vi "C to F.vi"(11 "Celsius":dbl) -> (3 "Fahrenheit":dbl)   [LabVIEW 2023, in "Simple Dual Mode Thermometer XControl.xctl"]
doc: "This VI converts degrees Celsius to degrees Fahrenheit."
uses:
  Simple Dual Mode Thermometer XControl.xctl
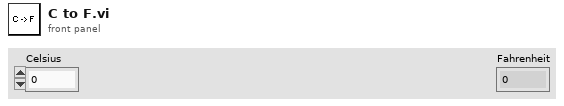
[diagram p1: front panel]
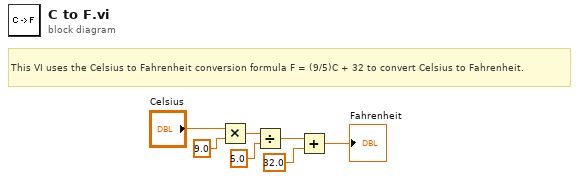
[diagram p0: block diagram]
diagram:
  # "This VI uses the Celsius to Fahrenheit conversion formula F = (9/5)C + 32 to convert Celsius to Fahrenheit."
  n1 = Multiply(x="Celsius", y=9.0) -> (x*y=w5:dbl)
  n2 = Divide(x=w5, y=5.0) -> (x/y=w3:dbl)
  n3 = Add(x=w3, y=32.0) -> (x+y=→"Fahrenheit":dbl)
